vi "Database_User_Edit.vi"(4 "error in":errorcluster, 5 "Language":T3, 6 "UserRight":T2, 7 "connection reference":T1) -> (0 "error out":errorcluster, 1 "Message":string, 3 "connection reference out":T1)   [LabVIEW 2015]
uses:
  CustomControl/Lang_Control.ctl
  CustomControl/UserRight.ctl
  <vilib>/addons/database/Connection.llb/Conn ObjectReference.ctl
  <vilib>/addons/database/NI_Database_API.lvlib
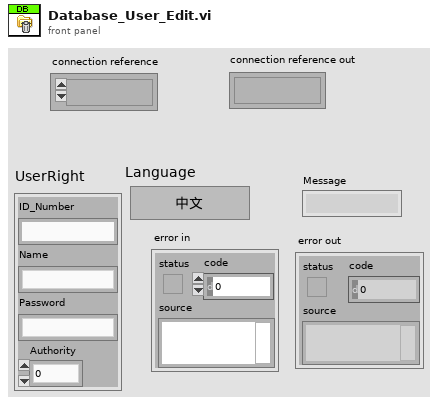
[diagram p1: front panel]
types:
  T1 = typedef "NI_Database_API.lvlib/Conn ObjectReference.ctl" = refnum<k1>
  T2 = typedef "UserRight.ctl" = cluster{"ID_Number":string, "Name":string, "Password":string, "Authority":i32}
  T3 = typedef "Lang_Control.ctl" = enum16{"中文", "English"}
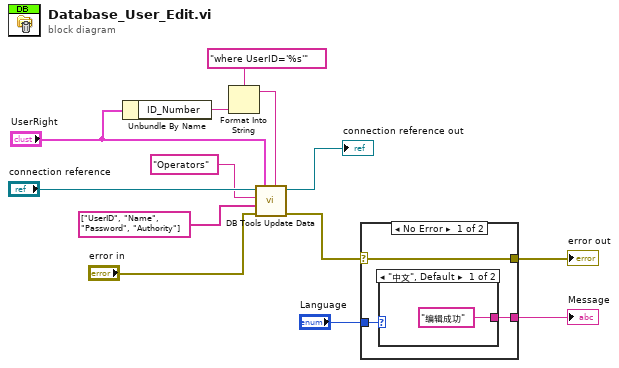
[diagram p0: block diagram]
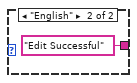
[diagram p2: hidden frame]
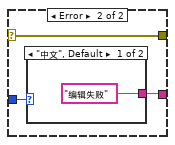
[diagram p3: hidden frame]
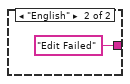
[diagram p4: hidden frame]
diagram:
  n1 = Unbundle By Name("UserRight") -> ("ID_Number"=w7:string)
  n2 = Format Into String(format string="where UserID='%s'", w7) -> (resulting string=w8:string)  [unwired: 2 in, 1 out]
  n3 = call <vilib>:"DB Tools Update Data.vi"("condition"=w8, "data"="UserRight", "error in (no error)"="error in", "columns"=string[] ["UserID", "Name", "Password", "Authority"], "table"="Operators", "connection reference"="connection reference") -> ("error out"=w6:errorcluster, "connection reference out"=→"connection reference out":T1)  [unwired: 4 in]
  n4 = case shown="No Error" w6 {
    selector: w6 -> [w16 w21]
    tunnel: [w16 w21] -> w13
    tunnel: [w15 w19] -> w12
    tunnel: "Language" -> [w14 w20]
    frame No Error {
      n5 = case shown="\"中文\", Default" w14 {
        tunnel: ["编辑成功" "Edit Successful"] -> w15
        frame "中文", Default {
        }
        frame "English" {
        }
      }
    }
    frame Error {
      n6 = case shown="\"中文\", Default" w20 {
        tunnel: ["编辑失败" "Edit Failed"] -> w19
        frame "中文", Default {
        }
        frame "English" {
        }
      }
    }
  }
  "error out" <- w13
  "Message" <- w12
